vi "CloseLoopScan.vi"() -> ()   [LabVIEW 2016]
uses:
  controls/Enum.ctl
  <vilib>/rvi/errors/niLvFpgaAdjustHostInterfaceError.vi
  <vilib>/regexp/Match Regular Expression.xnode
  <vilib>/rvi/interface/nirviReadWriteControl/nirviReadWriteControl.xnode
  controls/FPGAVIreferenceTypeDef.ctl
  FPGA Bitfiles/qnmController797_usbRio80MHz_1.lvbitx
  Course Project/support/Message Queue/Message Queue.lvlib
  NiFpgaLv.dll
panel:
  in  "Y":T1
  in  "X":T1 {"pGain" format="%#_3p"; "iGain" format="%#_3p"}
  in  "Close-Loop":bool
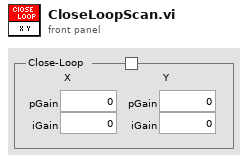
[diagram p1: front panel]
types:
  T1 = cluster{"pGain":fxp<+/-,20,4>, "iGain":fxp<+/-,20,1>}
  T2 = typedef "Message Queue.lvlib/All Message Queues.ctl" = cluster{"IU":refnum<queue>}
  T3 = typedef "Enum.ctl" = enum16{"Init", "Read", "Write"}
  T4 = typedef "FPGAVIreferenceTypeDef.ctl" = refnum<k20>
  T5 = cluster{"enable":bool, "setPoint":fxp<+/-,17,1>, "pGain":fxp<+/-,20,4>, "iGain":fxp<+/-,20,1>, "gainScale":i8}
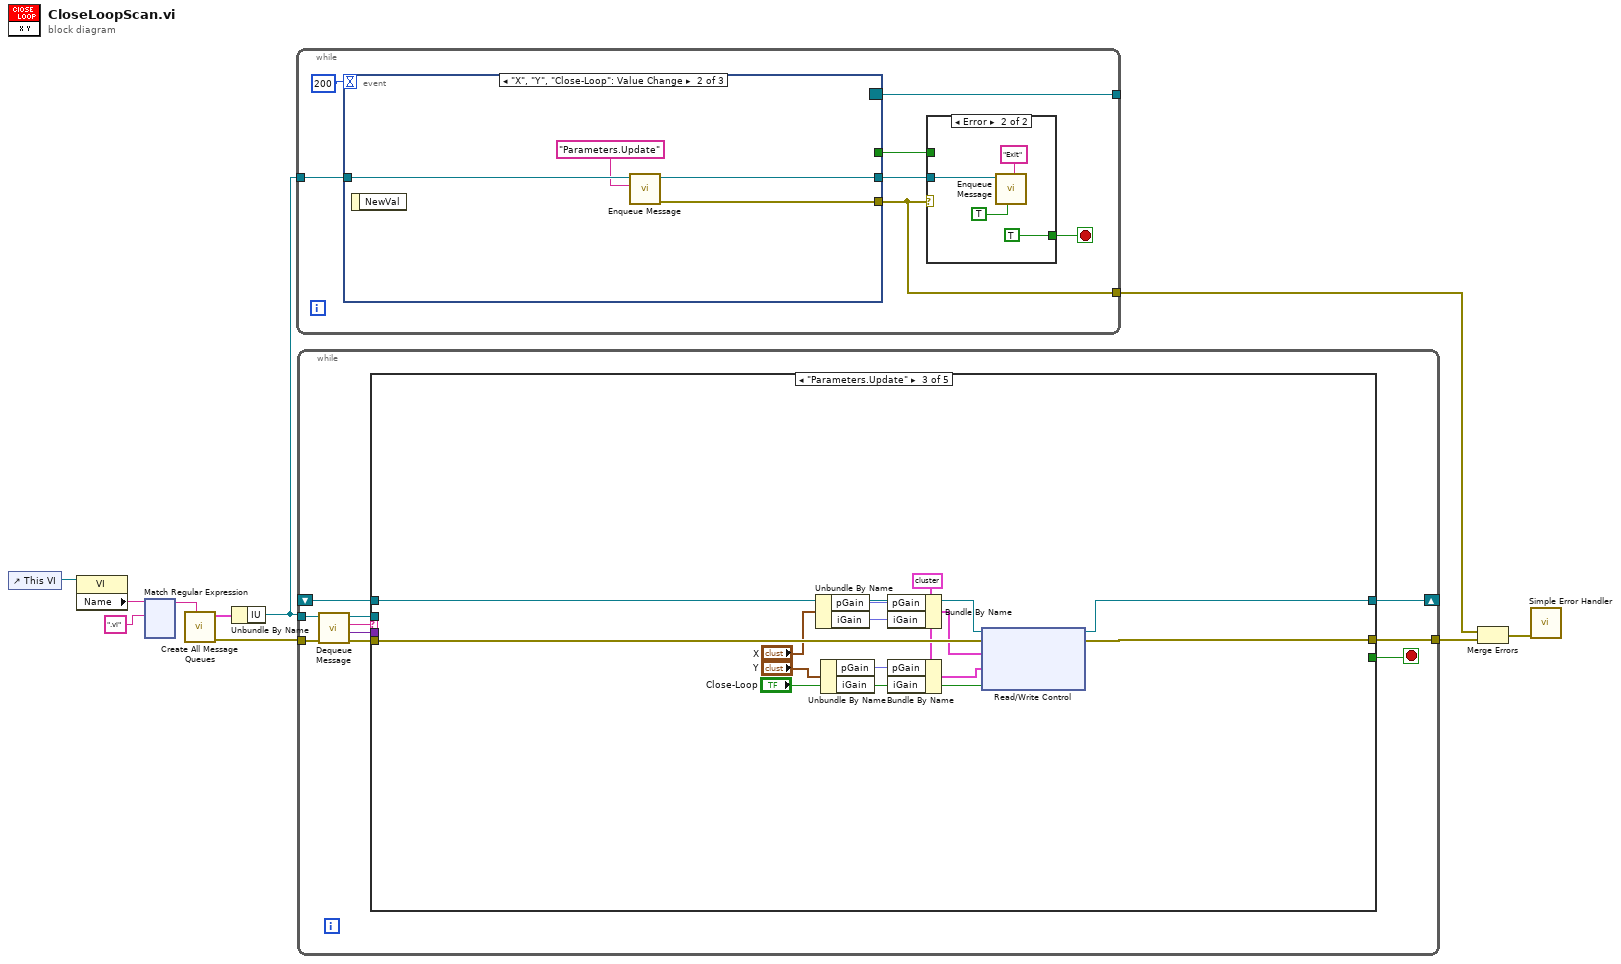
[diagram p0: block diagram]
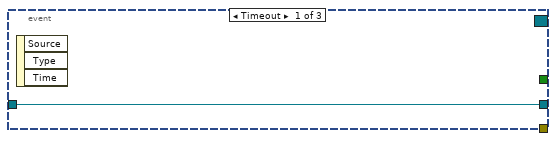
[diagram p3: hidden frame]
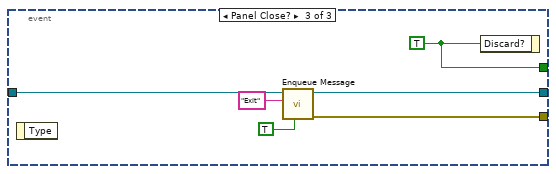
[diagram p4: hidden frame]
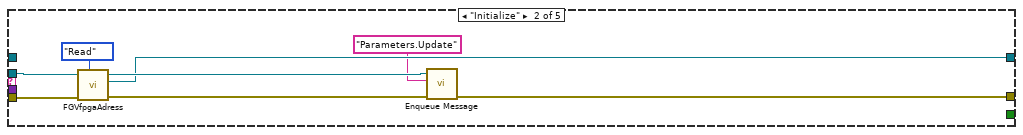
[diagram p6: hidden frame]
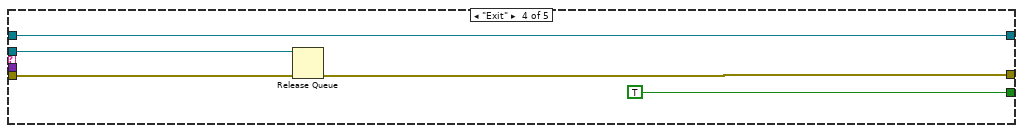
[diagram p7: hidden frame]
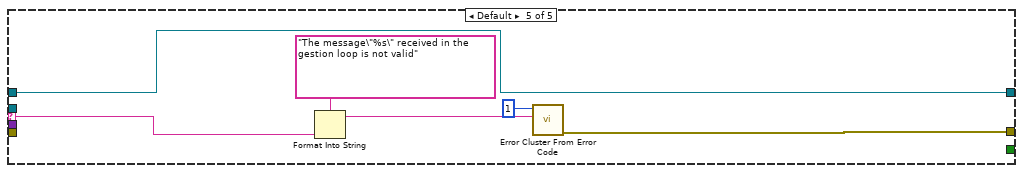
[diagram p8: hidden frame]
diagram:
  n1 = control-ref of="This VI"() -> (w4:refnum<vi>)
  n2 = property class="VI"(reference=w4) -> ("Name"=w3:string)  [unwired: 1 in, 2 out]
  n3 = xnode "Match Regular Expression"("input string"=w3, "regular expression"=".vi") -> ("before match"=w1:string)  [unwired: 4 in, 4 out]
  n4 = call "Create All Message Queues.vi"("QueueName"=w1) -> ("ErrorOut"=w8:errorcluster, "MessageQueueOut"=w10:T2)  [unwired: 9 in]
  n5 = Unbundle By Name(w10) -> ("IU"=w9:refnum<queue>)
  n6 = while {
    tunnel: w9 -> [w17]
    tunnel: [w13] -> w5
    tunnel: [w12] -> _
    stop <- w15 stop-if-true
    n7 = event shown="[1] \"X\", \"Y\", \"Close-Loop\": Value Change" {
      selector: _ -> [_ _ _]
      dyn-events: [_ _ _] -> w12
      timeout: 200 -> [_ _ _]
      tunnel: [_ _ w33] -> w16
      tunnel: w17 -> [w23 w27 w32]
      tunnel: [_ w24 w31] -> w13
      tunnel: [w23 w26 w30] -> w14
      event Timeout {
        n8 = event-data() -> ()  [unwired: 1 in, 3 out]
      }
      event "X", "Y", "Close-Loop": Value Change {
        n9 = event-data() -> ()  [unwired: 1 in, 1 out]
        n10 = call "Enqueue Message.vi"("Message"="Parameters.Update", "Queue"=w27) -> ("error out"=w24:errorcluster, "Queue dup."=w26:refnum<queue>)  [unwired: 8 in]
      }
      event Panel Close? {
        w33 = TRUE ("Rejeter ?")
        n11 = event-data() -> ()  [unwired: 1 in, 1 out]
        n12 = call "Enqueue Message.vi"("Prioritary message"=TRUE ("Message prioritaire ? (F)"), "Message"="Exit", "Queue"=w32) -> ("error out"=w31:errorcluster, "Queue dup."=w30:refnum<queue>)  [unwired: 7 in]
        n13 = event-data ("Event Filter Node")("Discard?"=w33) -> ()  [unwired: 1 in, 1 out]
      }
    }
    n14 = case shown="Error" w13 {
      tunnel: [w18 TRUE ("Rejeter ?")] -> w15
      tunnel: w16 -> [w18 _]
      tunnel: w14 -> [_ w21]
      frame No Error {
      }
      frame Error {
        n15 = call "Enqueue Message.vi"("Prioritary message"=TRUE ("Message prioritaire ? (F)"), "Message"="Exit", "Queue"=w21) -> ()  [unwired: 7 in, 2 out]
      }
    }
  }
  n16 = while {
    tunnel: w9 -> [w37]
    tunnel: w8 -> [w41]
    tunnel: [w42] -> w6
    shift-right: [w35] -> _
    shift-left: _ -> [w34]
    stop <- w43 stop-if-true
    n17 = call "Dequeue Message.vi"("entrée d'erreur (pas d'erreur)"=w41, "File d'attente de messages"=w37) -> ("sortie d'erreur"=w40:errorcluster, "Données de message"=w39:variant, "Message"=w36:string, "File d'attente de message dup."=w38:refnum<queue>)  [unwired: 6 in]
    n18 = case "Conditions des messages" shown="\"Parameters.Update\"" w36 {
      selector: w36 -> [_ _ _ _ w76]
      tunnel: w38 -> [_ w52 _ w71 _]
      tunnel: w40 -> [w45 w51 w66 w69 _]
      tunnel: [w45 w46 w65 w68 w74] -> w42
      tunnel: [_ _ _ TRUE _] -> w43
      tunnel: w39 -> [_ _ _ _ _]
      tunnel: [w44 w49 w63 w67 w72] -> w35
      tunnel: w34 -> [w44 _ w64 w67 w72]
      frame "--------- Initialization ---------" {
      }
      frame "Initialize" {
        n19 = call "FGVfpgaAdress.vi"("Enum"=Enum."Read", "error in"=w51) -> ("error out"=w47:errorcluster, "FPGA VI Reference Out"=w49:T4)  [unwired: 4 in, 4 out]
        n20 = call "Enqueue Message.vi"("error in"=w47, "Message"="Parameters.Update", "Queue"=w52) -> ("error out"=w46:errorcluster)  [unwired: 7 in, 1 out]
      }
      frame "Parameters.Update" {
        w54 = T5 {"enable"=TRUE, "setPoint"=0.0799407958984375, "pGain"=0.100006103515625, "iGain"=0.010000228881835938, "gainScale"=1} ("X")
        n21 = Unbundle By Name("X") -> ("pGain"=w60:fxp<+/-,20,4>, "iGain"=w59:fxp<+/-,20,1>)
        n22 = Unbundle By Name("Y") -> ("pGain"=w57:fxp<+/-,20,4>, "iGain"=w56:fxp<+/-,20,1>)
        n23 = Bundle By Name(cluster=w54, "pGain"=w60, "iGain"=w59) -> (w53:T5)
        n24 = Bundle By Name(cluster=w54, "pGain"=w57, "iGain"=w56) -> (w55:T5)
        n25 = xnode "Read/Write Control"("FPGA VI Reference In"=w64, "error in"=w66, "se.p.x.fbParams"=w53, "se.p.y.fbParams"=w55, "se.p.closedLoop"="Close-Loop") -> ("FPGA VI Reference Out"=w63:T4, "error out"=w65:errorcluster)
      }
      frame "Exit" {
        n26 = Release Queue(queue=w71, error in (no error)=w69) -> (error out=w68:errorcluster)  [unwired: 1 in, 2 out]
      }
      frame Default {
        n27 = Format Into String(format string="The message\"%s\" received in the gestion loop is not valid" ("Texte de message d'erreur inconnu"), w76) -> (resulting string=w73:string)  [unwired: 2 in, 1 out]
        n28 = call <vilib>:"Error Cluster From Error Code.vi"("error message (\"\")"=w73, "error code (0)"=1 ("code d'erreur (0)")) -> ("error out"=w74:errorcluster)  [unwired: 7 in]
      }
    }
  }
  n29 = Merge Errors(w5, w6) -> (w7:errorcluster)
  n30 = call <vilib>:"Simple Error Handler.vi"("error in (no error)"=w7) -> ()  [unwired: 4 in, 5 out]
